vi "Main Abstraction Level 3.vi"() -> ()   [LabVIEW 2023]
doc: "This is one of the levels of abstract design along the timeline leading to the goal of a complete measurement application."
uses:
  messages/MeasureAndLogMessage.lvclass/MeasureAndLogMessage.ctl
  <extravilib>/ChannelInstances/Lossy Stream-a[.](wfm(dbl))/Read With Abort.vi
  <extravilib>/ChannelInstances/Stream-str/Read With Abort.vi
  <extravilib>/ChannelInstances/Messenger-class'MeasureAndLogMessage'/Write With Abort.vi
  <extravilib>/ChannelInstances/Lossy Stream-a[.](wfm(dbl))/EndpointRead.vi
  <extravilib>/ChannelInstances/Stream-str/EndpointRead.vi
  <extravilib>/ChannelInstances/Stream-a[.](wfm(dbl))/Instantiate.vi
  <extravilib>/ChannelInstances/Tag-path/Instantiate.vi
  <extravilib>/ChannelInstances/Stream-str/Instantiate.vi
  <extravilib>/ChannelInstances/Stream-str/)Channel.vi
  <resource>/ChannelSupport/_ChannelSupport/WaitIfNeeded.vi
  <extravilib>/ChannelInstances/Lossy Stream-a[.](wfm(dbl))/Instantiate.vi
  <extravilib>/ChannelInstances/Lossy Stream-a[.](wfm(dbl))/)Channel.vi
  <extravilib>/ChannelInstances/Messenger-class'MeasureAndLogMessage'/Instantiate.vi
  <extravilib>/ChannelInstances/Messenger-class'MeasureAndLogMessage'/Endpoint.vi
  messages/MeasureAndLogMessage.lvclass
  <extravilib>/ChannelInstances/Stream-str.lvlib
  <extravilib>/ChannelInstances/Lossy Stream-a[.](wfm(dbl)).lvlib
  <extravilib>/ChannelInstances/Messenger-class'MeasureAndLogMessage'.lvlib
panel:
  in  "Exit flag":bool
  in  "Record":bool
  in  "Stop":bool
  out "Data":waveform(dbl)[](graph)
  out "Status":string
  in  "Settings":bool
  in  "Start":bool
  in  "Exit":bool
  # "Continuous Measurement Data Logger"
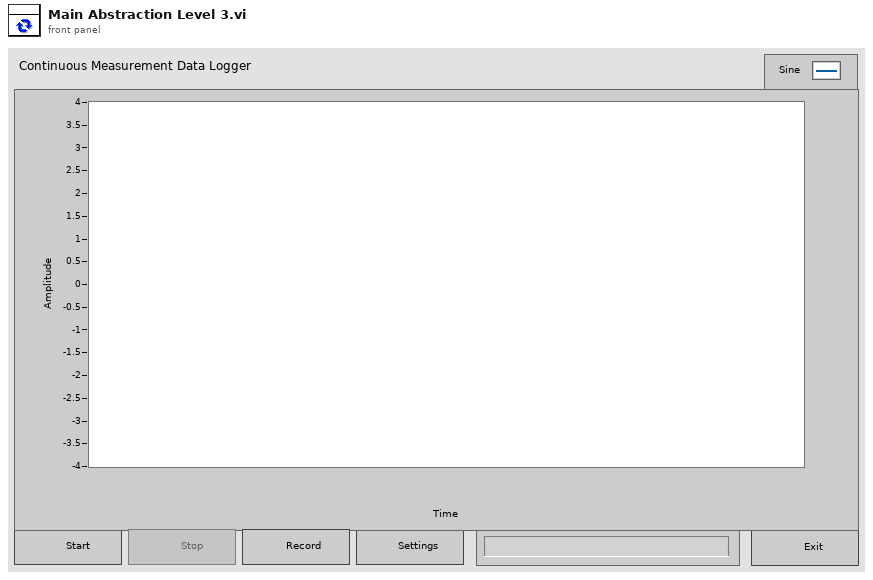
[diagram p1: front panel]
types:
  T1 = typedef "Measure and Log Settings.ctl" = cluster{"sample rate":dbl, "input range":dbl, "logfile path":path, "Simulated Signal":cluster{"signal type":T2, "frequency":dbl, "amplitude":dbl}}
  T2 = typedef "Simulated Signal Type.ctl" = enum16{"Sine Wave", "Square Wave with Noise"}
  T3 = enum8{"Enabled", "Disabled", "Disabled and Grayed Out"}
  T4 = typedef "Messenger-class'MeasureAndLogMessage'.lvlib/))Channel.ctl" = refnum<queue>
  T5 = typedef "Stream-a[.](wfm(dbl)).lvlib/)Channel.ctl" = refnum<queue>
  T6 = typedef "Tag-path.lvlib/))Channel.ctl" = refnum<queue>
  T7 = typedef "Stream-str.lvlib/)Channel.ctl" = refnum<queue>
  T8 = typedef "Lossy Stream-a[.](wfm(dbl)).lvlib/)Channel.ctl" = refnum<queue>
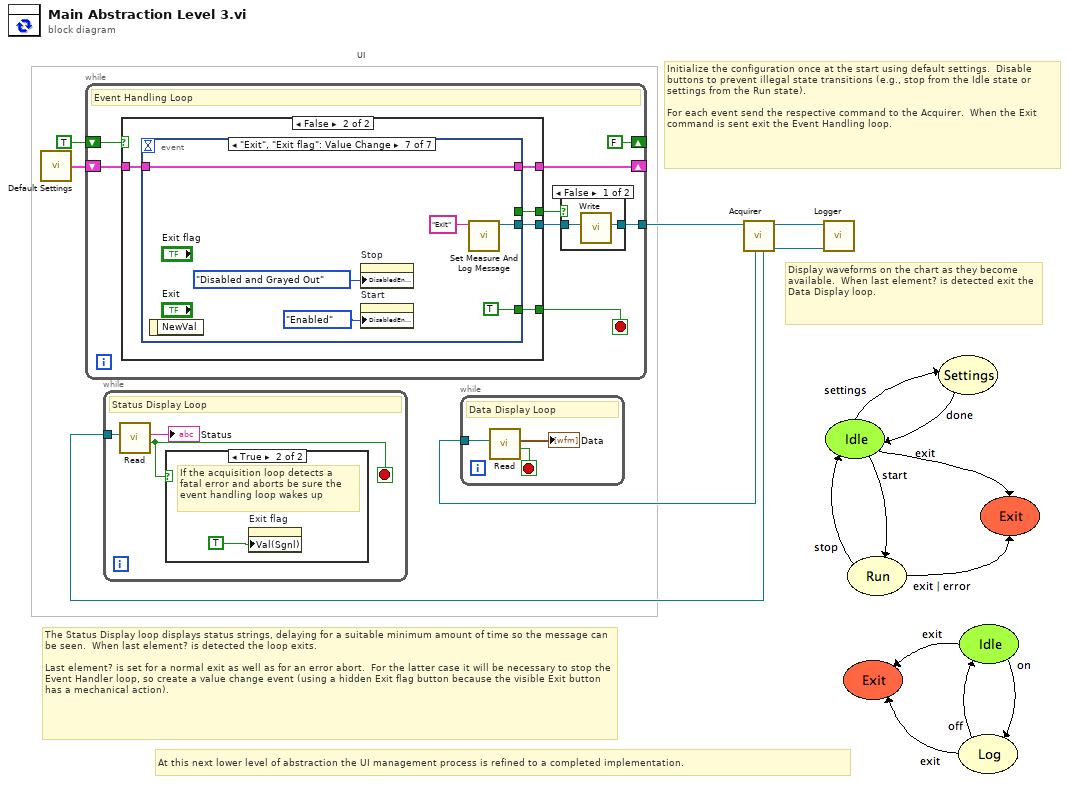
[diagram p0: block diagram]
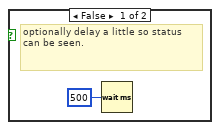
[diagram p2: hidden frame]
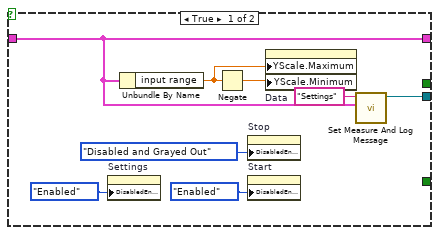
[diagram p3: hidden frame]
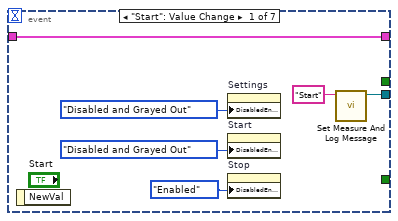
[diagram p4: hidden frame]
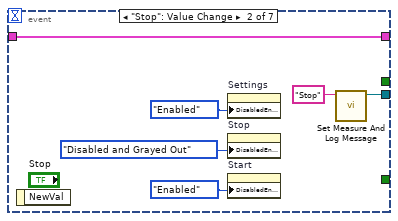
[diagram p5: hidden frame]
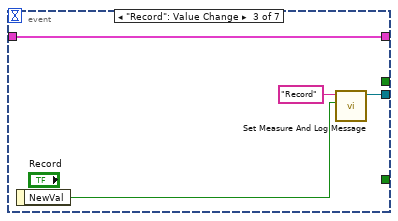
[diagram p6: hidden frame]
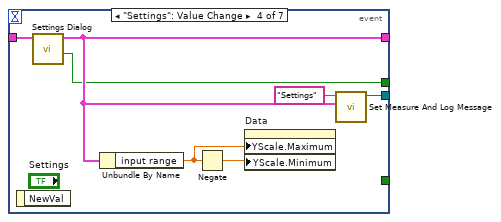
[diagram p7: hidden frame]
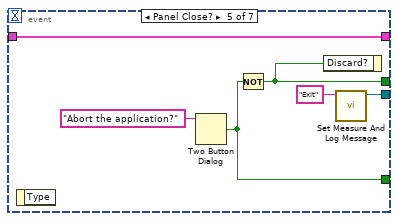
[diagram p8: hidden frame]
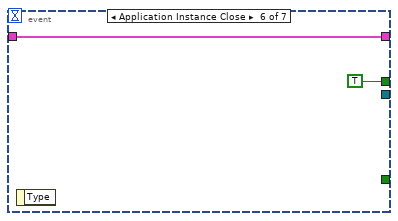
[diagram p9: hidden frame]
diagram:
  # "At this next lower level of abstraction the UI management process is refined to a completed implementation."
  # "Display waveforms on the chart as they become available.  When last element? is detected exit the Data Display loop."
  # "Initialize the configuration once at the start using default settings.  Disable buttons to prevent illegal state transitions (e.g., stop from the Idle state or settings from the Run state).\n\nFor each event send the respective command to the Acquirer.  When the Exit command is sent exit the Event Handling loop."
  # "UI"
  # "The Status Display loop displays status strings, delaying for a suitable minimum amount of time so the message can be seen.  When last element? is detected the loop exits.  \n\nLast element? is set for a normal exit as well as for an error abort.  For the latter case it will be necessary to stop the Event Handler loop, so create a value change event (using a hidden Exit flag button because the visible Exit button has a mechanical action)."
  n1 = call "Default Settings.vi"() -> ("default settings"=w6:T1)
  n2 = while {
    tunnel: [w12] -> w7
    shift-right: [w14] -> _
    shift-left: w6 -> [w13]
    shift-right: [FALSE] -> _
    shift-left: TRUE -> [w8]
    stop <- w15 stop-if-true
    # "Event Handling Loop"
    n3 = case shown="False" w8 {
      tunnel: [_ w28] -> w15
      tunnel: [w22 w27] -> w14
      tunnel: w13 -> [w22 w26]
      tunnel: [w18 w25] -> w11
      tunnel: [_ w24] -> w10
      frame True {
        n4 = property on="Settings" class="Bool"("DisabledEnum"=T3."Enabled" ("Disabled")) -> ()  [unwired: 2 in, 2 out]
        n5 = Unbundle By Name(w22) -> ("input range"=w16:dbl)
        n6 = Negate(x=w16) -> (-x=w17:dbl)
        n7 = property on="Stop" class="Bool"("DisabledEnum"=T3."Disabled and Grayed Out" ("Disabled")) -> ()  [unwired: 2 in, 2 out]
        n8 = property on="Start" class="Bool"("DisabledEnum"=T3."Enabled" ("Disabled")) -> ()  [unwired: 2 in, 2 out]
        n9 = property on="Data" class="WFChart (strict)"("YScale.Maximum"=w16, "YScale.Minimum"=w17) -> ()  [unwired: 2 in, 2 out]
        n10 = call "Set Measure And Log Message.vi"("args"=w22, "command"="Settings") -> ("MyMessage"=w18:refnum<class "MeasureAndLogMessage.lvclass">)  [unwired: 9 in]
      }
      frame False {
        n11 = event shown="[6] \"Exit\", \"Exit flag\": Value Change" {
          selector: _ -> [_ _ _ _ _ _ _]
          dyn-events: _ -> [_ _ _ _ _ _ _]
          timeout: _ -> [_ _ _ _ _ _ _]
          tunnel: [_ _ _ _ w53 _ TRUE] -> w28
          tunnel: [w30 w36 w42 w50 w56 w59 w61] -> w27
          tunnel: w26 -> [w30 w36 w42 w51 w56 w59 w61]
          tunnel: [w29 w35 w41 w49 w54 _ w60] -> w25
          tunnel: [_ _ _ w47 w52 TRUE ("cancelled") _] -> w24
          event "Start": Value Change {
            n12 = event-data() -> ()  [unwired: 1 in, 1 out]
            n13 = property on="Settings" class="Bool"("DisabledEnum"=T3."Disabled and Grayed Out" ("Disabled")) -> ()  [unwired: 2 in, 2 out]
            n14 = property on="Start" class="Bool"("DisabledEnum"=T3."Disabled and Grayed Out" ("Disabled")) -> ()  [unwired: 2 in, 2 out]
            n15 = property on="Stop" class="Bool"("DisabledEnum"=T3."Enabled" ("Disabled")) -> ()  [unwired: 2 in, 2 out]
            n16 = call "Set Measure And Log Message.vi"("command"="Start") -> ("MyMessage"=w29:refnum<class "MeasureAndLogMessage.lvclass">)  [unwired: 10 in]
          }
          event "Stop": Value Change {
            n17 = event-data() -> ()  [unwired: 1 in, 1 out]
            n18 = property on="Settings" class="Bool"("DisabledEnum"=T3."Enabled" ("Disabled")) -> ()  [unwired: 2 in, 2 out]
            n19 = property on="Stop" class="Bool"("DisabledEnum"=T3."Disabled and Grayed Out" ("Disabled")) -> ()  [unwired: 2 in, 2 out]
            n20 = property on="Start" class="Bool"("DisabledEnum"=T3."Enabled" ("Disabled")) -> ()  [unwired: 2 in, 2 out]
            n21 = call "Set Measure And Log Message.vi"("command"="Stop") -> ("MyMessage"=w35:refnum<class "MeasureAndLogMessage.lvclass">)  [unwired: 10 in]
          }
          event "Record": Value Change {
            n22 = event-data() -> ("NewVal"=w43:bool)  [unwired: 1 in]
            n23 = call "Set Measure And Log Message.vi"("args"=w43, "command"="Record") -> ("MyMessage"=w41:refnum<class "MeasureAndLogMessage.lvclass">)  [unwired: 9 in]
          }
          event "Settings": Value Change {
            n24 = event-data() -> ()  [unwired: 1 in, 1 out]
            n25 = call "Settings Dialog.vi"("settings in"=w51) -> ("cancelled"=w47:bool, "settings out"=w50:T1)  [unwired: 9 in]
            n26 = Unbundle By Name(w50) -> ("input range"=w45:dbl)
            n27 = Negate(x=w45) -> (-x=w46:dbl)
            n28 = property on="Data" class="WFChart (strict)"("YScale.Maximum"=w45, "YScale.Minimum"=w46) -> ()  [unwired: 2 in, 2 out]
            n29 = call "Set Measure And Log Message.vi"("args"=w50, "command"="Settings") -> ("MyMessage"=w49:refnum<class "MeasureAndLogMessage.lvclass">)  [unwired: 9 in]
          }
          event Panel Close? {
            n30 = event-data() -> ()  [unwired: 1 in, 1 out]
            n31 = Two Button Dialog(message="Abort the application?") -> (T button?=w53:bool)  [unwired: 2 in]
            n32 = Not(x=w53) -> (.not. x?=w52:bool)
            n33 = event-data("Discard?"=w52) -> ()  [unwired: 1 in, 1 out]
            n34 = call "Set Measure And Log Message.vi"("command"="Exit") -> ("MyMessage"=w54:refnum<class "MeasureAndLogMessage.lvclass">)  [unwired: 10 in]
          }
          event Application Instance Close {
            n35 = event-data() -> ()  [unwired: 1 in, 1 out]
          }
          event "Exit", "Exit flag": Value Change {
            n36 = event-data() -> ()  [unwired: 1 in, 1 out]
            n37 = property on="Stop" class="Bool"("DisabledEnum"=T3."Disabled and Grayed Out" ("Disabled")) -> ()  [unwired: 2 in, 2 out]
            n38 = property on="Start" class="Bool"("DisabledEnum"=T3."Enabled" ("Disabled")) -> ()  [unwired: 2 in, 2 out]
            n39 = call "Set Measure And Log Message.vi"("command"="Exit") -> ("MyMessage"=w60:refnum<class "MeasureAndLogMessage.lvclass">)  [unwired: 10 in]
          }
        }
      }
    }
    n40 = case shown="False" w10 {
      tunnel: [w67 _] -> w12
      tunnel: w11 -> [w66 _]
      frame False {
        n41 = call <extravilib>:"Write.vi"("element"=w66) -> ("channel"=w67:T4)  [unwired: 8 in, 2 out]
      }
      frame True {
      }
    }
  }
  n42 = call "Acquirer.vi"("command stream"=w7) -> ("wfm data stream"=w2:T5, "file path tag"=w3:T6, "status stream"=w4:T7, "wfm data lossy stream"=w5:T8)  [unwired: 7 in]
  n43 = while {
    tunnel: w4 -> [w70]
    stop <- w68 stop-if-true
    # "Status Display Loop"
    n44 = call <extravilib>:"Read.vi"("channel"=w70) -> ("last element?"=w68:bool, "element"=→"Status":string)  [unwired: 6 in, 3 out]
    n45 = case shown="True" w68 {
      frame False {
        # "optionally delay a little so status can be seen."
        n46 = Wait (ms)(milliseconds to wait=u32 500) -> ()  [unwired: 1 out]
      }
      frame True {
        # "If the acquisition loop detects a fatal error and aborts be sure the event handling loop wakes up"
        n47 = property on="Exit flag" class="Bool (strict)"("Val(Sgnl)"=TRUE) -> ()  [unwired: 2 in, 2 out]
      }
    }
  }
  n48 = while {
    tunnel: w5 -> [w73]
    stop <- w75 stop-if-true
    # "Data Display Loop"
    n49 = call <extravilib>:"Read.vi"("channel"=w73) -> ("last element?"=w75:bool, "element"=→"Data":waveform(dbl)[])  [unwired: 5 in, 4 out]
  }
  n50 = call "Logger.vi"("wfm data stream"=w2, "file path tag"=w3) -> ()  [unwired: 9 in, 1 out]
